vi "Write Desired Temperature.vi"(10 "待维持的温度":dbl=75.0, 11 "冷却器输入":refnum<class "Cooler.lvclass">) -> (3 "冷却器输出":refnum<class "Cooler.lvclass">)   [LabVIEW 2013, in "Cooler.lvlib" / "Cooler.lvclass"]
doc: "写入系统需要维持的温度。"
uses:
  Cooler.lvclass
  Level Controller/Level Controller/Deadband.ctl
  Level Controller/Level Controller/Level Controller.lvclass
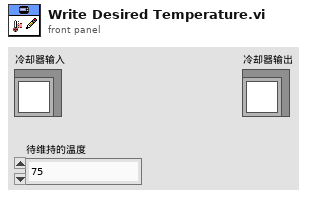
[diagram p1: front panel]
types:
  T1 = typedef "Level Controller.lvlib/Level Controller.lvclass/Deadband.ctl" = cluster{"Low":dbl, "High":dbl}
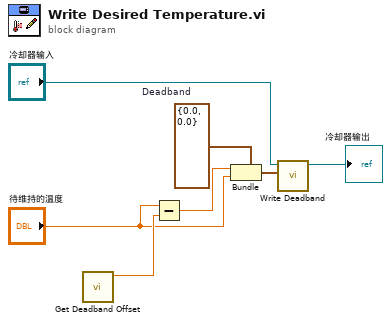
[diagram p0: block diagram]
diagram:
  w1 = T1 {"Low"=0.0, "High"=0.0}  # Deadband
  n1 = call "Get Deadband Offset.vi"() -> ("死区偏移"=w7:dbl)  [unwired: 11 in]
  n2 = Subtract(x="待维持的温度", y=w7) -> (x-y=w6:dbl)
  n3 = Bundle(cluster=w1, "Low"=w6, "High"="待维持的温度") -> (w2:T1)
  n4 = call "Write Deadband.vi"("死区"=w2, "水位控制器输入"="冷却器输入") -> ("水位控制器输出"=→"冷却器输出":refnum<class "Cooler.lvclass">)  [unwired: 8 in, 1 out]
